vi "BLM Wait for Move.vi"(5 "error in (no error)":errorcluster, 7 "Motor Address":string="0", 8 "PORT Address":refnum<visa-resource-name>) -> (0 "error out":errorcluster, 2 "Motor moves":bool, 3 "PORT Address 2":refnum<visa-resource-name>)   [LabVIEW 2019]
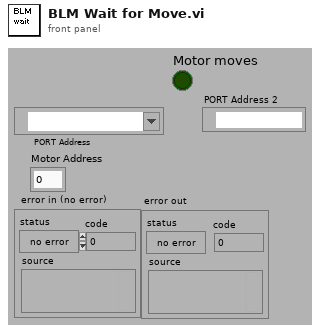
[diagram p1: front panel]
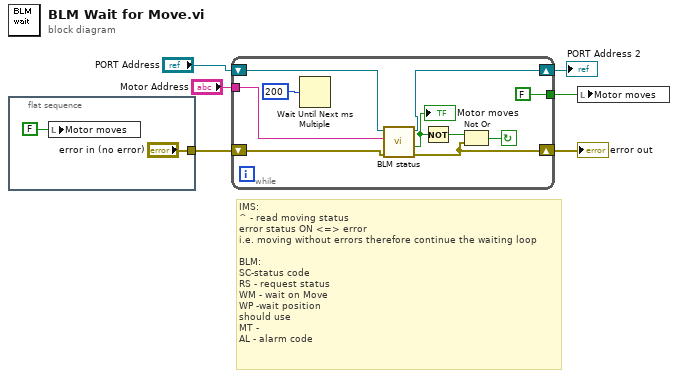
[diagram p0: block diagram]
diagram:
  # "IMS:\n^ - read moving status\nerror status ON <=> error\ni.e. moving without errors therefore continue the waiting loop\n\nBLM:\nSC-status code\nRS - request status\nWM - wait on Move\nWP -wait position\nshould use\nMT - \nAL - alarm code"
  n1 = flat-sequence {
    tunnel: ["error in (no error)"] -> w5
    frame #0 {
      n2 = local write "Motor moves"(FALSE ("Motor moves")) -> ()
    }
  }
  n3 = while {
    shift-left: w5 -> [w15]
    shift-right: [w12] -> w6
    tunnel: "Motor Address" -> [w13]
    tunnel: [FALSE ("Read Echo?")] -> w3
    shift-right: [w9] -> w1
    shift-left: "PORT Address" -> [w10]
    stop <- w18 continue-if-true
    n4 = Wait Until Next ms Multiple(millisecond multiple=u32 200) -> ()  [unwired: 1 out]
    n5 = call "BLM status.vi"("error in (no error)"=w15, "Motor Address"=w13, "Port Address"=w10) -> ("error out"=w12:errorcluster, "Motor is moving"=w14:bool, "Port Address Out"=w9:refnum<visa-resource-name>)  [unwired: 2 in]
    "Motor moves" <- w14
    n6 = Not(x=w14) -> (.not. x?=w17:bool)
    n7 = Not Or(1:w12, 2:w17) -> (0:w18:bool)
  }
  "error out" <- w6
  "PORT Address 2" <- w1
  n8 = local write "Motor moves"(w3) -> ()
